vi "OIL_FILLING.vi"(8 "error in (no error)":errorcluster, 11 "Stand in":refnum<class "Stand.lvclass">) -> (0 "error out":errorcluster, 3 "Stand out":refnum<class "Stand.lvclass">)   [LabVIEW 2019, in "Stand.lvclass"]
uses:
  Stand.lvclass
  AI_class/AI.lvclass
  Sig_DI_Simple_class/Sig_DI_Simple.lvclass
  TypeDef/State OIL_FILLING.ctl
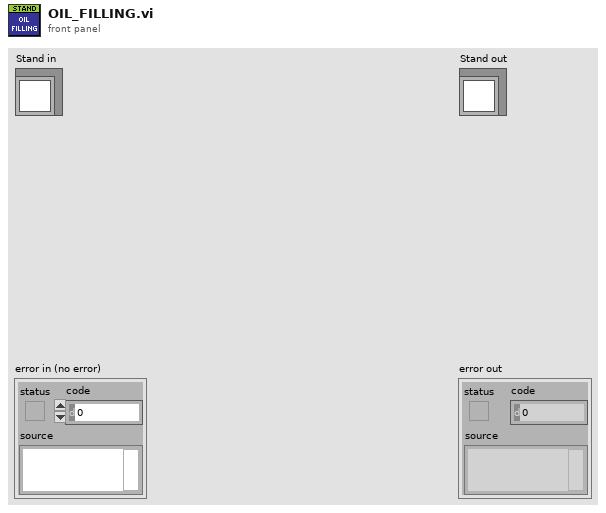
[diagram p1: front panel]
types:
  T1 = typedef "State OIL_FILLING.ctl" = enum16{"NOT READY", "READY", "TURNING ON", "ON", "TURNING OFF"}
  T2 = typedef "AI_Data.ctl" = cluster{"Raw":dbl, "Scaled":dbl, "OutOfRangeMax":bool, "OutOfRangeMin":bool, "HIHI":bool, "HI":bool, "LO":bool, "LOLO":bool, "OutOfRangeMax_val":dbl, "OutOfRangeMin_val":dbl, "HIHI_val":dbl, "HI_val":dbl, "LO_val":dbl, "LOLO_val":dbl}
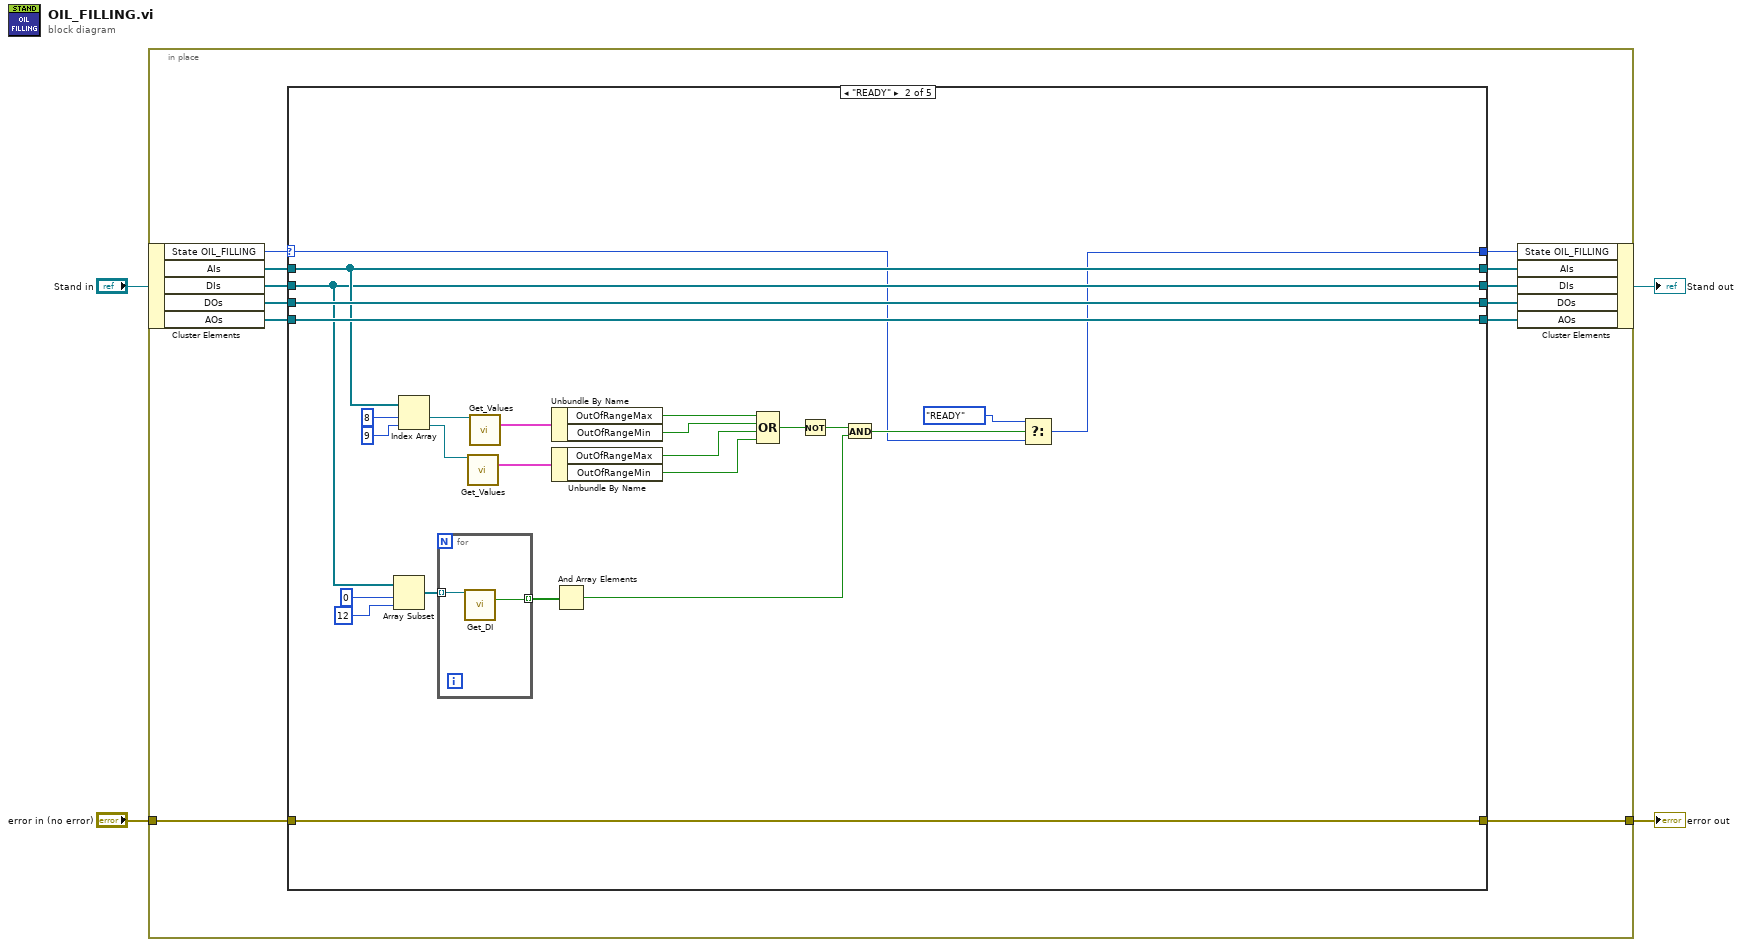
[diagram p0: block diagram]
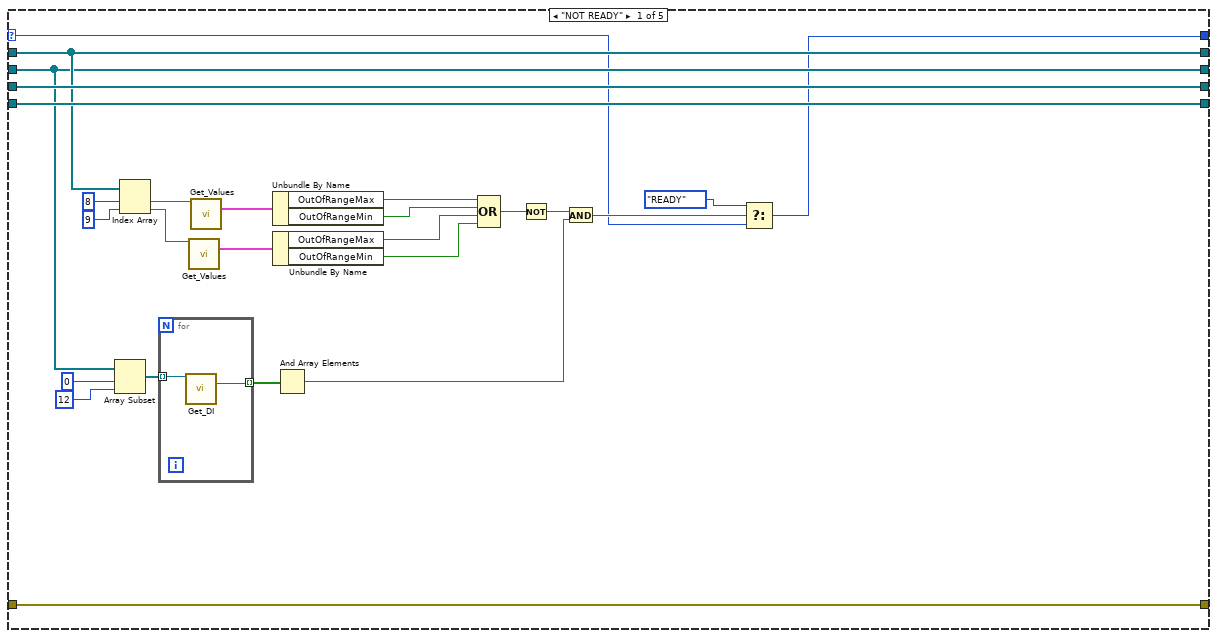
[diagram p2: hidden frame]
diagram:
  n1 = in-place {
    in-place-border: [w15] -> w2
    in-place-border: "error in (no error)" -> [w14]
    n2 = in-place-cluster #1("Stand in") -> ("State OIL_FILLING"=w16:T1, "AIs"=w11:refnum<class "AI.lvclass">[], "DIs"=w9:refnum<class "Sig_DI_Simple.lvclass">[], "DOs"=w7:refnum<class "DO.lvclass">[], "AOs"=w5:refnum<class "Sig_AO.lvclass">[])
    n3 = case shown="\"READY\"" w16 {
      selector: w16 -> [w19 w47 w73 w79 w85]
      tunnel: [w42 w70 w78 w84 w90] -> w15
      tunnel: w14 -> [w42 w70 w78 w84 w90]
      tunnel: [w17 w45 w73 w79 w85] -> w13
      tunnel: [w39 w67 w77 w83 w89] -> w12
      tunnel: w11 -> [w39 w67 w77 w83 w89]
      tunnel: [w28 w56 w76 w82 w88] -> w10
      tunnel: w9 -> [w28 w56 w76 w82 w88]
      tunnel: [w41 w69 w75 w81 w87] -> w8
      tunnel: w7 -> [w41 w69 w75 w81 w87]
      tunnel: [w40 w68 w74 w80 w86] -> w6
      tunnel: w5 -> [w40 w68 w74 w80 w86]
      frame "NOT READY" {
        n4 = Array Subset(array=w28, index=0, length=12) -> (w25:refnum<class "Sig_DI_Simple.lvclass">[])
        n5 = Index Array(array=w39, index #1=8 ("index"), index #2=9 ("index")) -> (element #1=w38:refnum<class "AI.lvclass">, element #2=w35:refnum<class "AI.lvclass">)
        n6 = for {
          tunnel: w25 -> [w44] mode=indexing
          tunnel: [w43] -> w24 mode=indexing
          n7 = call "Get_DI.vi"("reference in"=w44) -> ("DI"=w43:bool)  [unwired: 14 in]
        }
        n8 = call "Get_Values.vi"("reference in"=w35) -> ("Data"=w33:T2)  [unwired: 14 in]
        n9 = call "Get_Values.vi"("reference in"=w38) -> ("Data"=w34:T2)  [unwired: 14 in]
        n10 = Unbundle By Name(w34) -> ("OutOfRangeMax"=w32:bool, "OutOfRangeMin"=w31:bool)
        n11 = Unbundle By Name(w33) -> ("OutOfRangeMax"=w30:bool, "OutOfRangeMin"=w29:bool)
        n12 = And Array Elements(Boolean array=w24) -> (logical AND=w21:bool)
        n13 = Compound Arithmetic op=OR(w32, w31, w30, w29) -> (w23:bool)
        n14 = Not(x=w23) -> (.not. x?=w22:bool)
        n15 = And(x=w22, y=w21) -> (x .and. y?=w20:bool)
        n16 = Select(t=State_OIL_FILLING."READY", s=w20, f=w19) -> (s? t:f=w17:T1)
      }
      frame "READY" {
        n17 = Array Subset(array=w56, index=0, length=12) -> (w53:refnum<class "Sig_DI_Simple.lvclass">[])
        n18 = Index Array(array=w67, index #1=8 ("index"), index #2=9 ("index")) -> (element #1=w66:refnum<class "AI.lvclass">, element #2=w63:refnum<class "AI.lvclass">)
        n19 = for {
          tunnel: w53 -> [w72] mode=indexing
          tunnel: [w71] -> w52 mode=indexing
          n20 = call "Get_DI.vi"("reference in"=w72) -> ("DI"=w71:bool)  [unwired: 14 in]
        }
        n21 = call "Get_Values.vi"("reference in"=w63) -> ("Data"=w61:T2)  [unwired: 14 in]
        n22 = call "Get_Values.vi"("reference in"=w66) -> ("Data"=w62:T2)  [unwired: 14 in]
        n23 = Unbundle By Name(w62) -> ("OutOfRangeMax"=w60:bool, "OutOfRangeMin"=w59:bool)
        n24 = Unbundle By Name(w61) -> ("OutOfRangeMax"=w58:bool, "OutOfRangeMin"=w57:bool)
        n25 = And Array Elements(Boolean array=w52) -> (logical AND=w49:bool)
        n26 = Compound Arithmetic op=OR(w60, w59, w58, w57) -> (w51:bool)
        n27 = Not(x=w51) -> (.not. x?=w50:bool)
        n28 = And(x=w50, y=w49) -> (x .and. y?=w48:bool)
        n29 = Select(t=State_OIL_FILLING."READY", s=w48, f=w47) -> (s? t:f=w45:T1)
      }
      frame "TURNING ON" {
      }
      frame "ON" {
      }
      frame "TURNING OFF" {
      }
    }
    n30 = in-place-cluster #1("State OIL_FILLING"=w13, "AIs"=w12, "DIs"=w10, "DOs"=w8, "AOs"=w6) -> (→"Stand out":refnum<class "Stand.lvclass">)
  }
  "error out" <- w2
